vi "Test enum to string.vi"() -> ()   [LabVIEW 2019]
uses:
  Instrument/Typedefs/Instrument.Commands--Enum.ctl
  a588928e-b79e-47fd-8b2f-27266a521fd2.vi
  97061c39-901d-49d9-9773-b5b8f94cdda8.vi
  a46d76b3-4efe-4f1f-b7b6-6a97a4340745.vi
  b95be834-838a-46c0-a103-ccf79b46d759.vi
  <vilib>/Utility/Data Type/Get Type Information.vi
  <vilib>/Utility/Data Type/Get Numeric Information.vi
  <userlib>/_OpenG.lib/lvdata/lvdata.llb/Unwrap VVariant__ogtk.vi
  Instrument/Instrument.lvclass
panel:
  out "string to variant to string":string[](array[string])
  out "enum to variant to string":string[](array[string])
  out "string to string":string[](array[string])
  out "enum to string":string[](array[string])
  out "string to variant to string":string
  out "enum to variant to string":string
  out "enum to string":string
  out "string to string":string
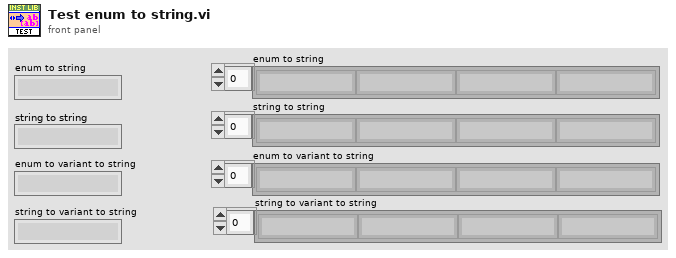
[diagram p1: front panel]
types:
  T1 = typedef "Instrument.lvclass/Instrument.Commands--Enum.ctl" = enum16{"ACK", "HELP", "IDN", "getAll", "getAllData"}
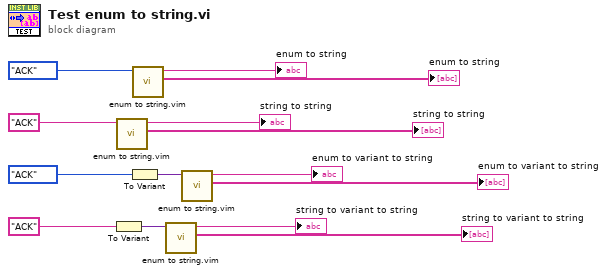
[diagram p0: block diagram]
diagram:
  n1 = To Variant(anything="ACK") -> (Variant=w5:variant)
  n2 = call "enum to string.vim"("enum in"="ACK") -> ("strings out"=→"string to string":string[], "string out"=→"string to string":string)  [unwired: 9 in]
  n3 = To Variant(anything=Instrument.Commands--Enum."ACK" ("PublicCommands")) -> (Variant=w6:variant)
  n4 = call "enum to string.vim"("enum in"=Instrument.Commands--Enum."ACK" ("PublicCommands")) -> ("strings out"=→"enum to string":string[], "string out"=→"enum to string":string)  [unwired: 9 in]
  n5 = call "enum to string.vim"("enum in"=w5) -> ("strings out"=→"string to variant to string":string[], "string out"=→"string to variant to string":string)  [unwired: 9 in]
  n6 = call "enum to string.vim"("enum in"=w6) -> ("strings out"=→"enum to variant to string":string[], "string out"=→"enum to variant to string":string)  [unwired: 9 in]
